vi "Update User Interface.vi"(8 "error in (no error)":errorcluster, 11 "Model in":refnum<class "Model.lvclass">) -> (0 "error out":errorcluster, 3 "Model out":refnum<class "Model.lvclass">)   [LabVIEW 2018, in "Model.lvlib" / "Model.lvclass"]
uses:
  Model.lvclass
  Model.lvclass/Model.ctl
  Interface Messages/Update VI List Msg/Update VI List Msg.lvclass/Update VI List Msg.ctl
  <vilib>/ActorFramework/Message Enqueuer/Message Enqueuer.lvclass/Message Enqueuer.ctl
  <vilib>/ActorFramework/Message Enqueuer/Enqueue.vi
  Interface Messages/Update VI List Msg/Update VI List Msg.lvclass
  C:/Program Files/National Instruments/LabVIEW 2018/vi.lib/ActorFramework/Message/Message.lvclass
  <vilib>/ActorFramework/Message Priority Queue/Priority Enqueue.vi
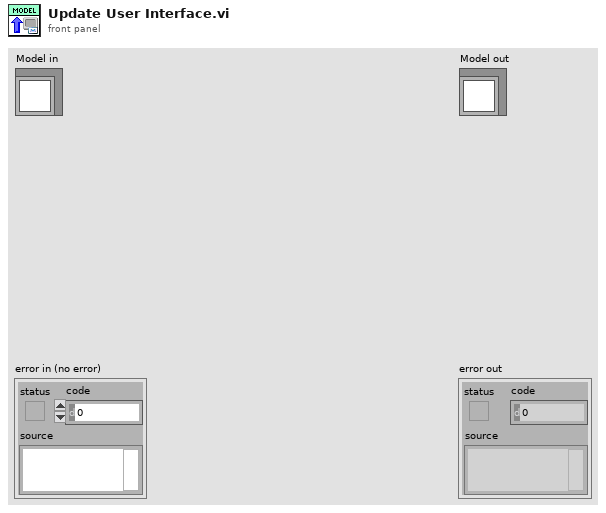
[diagram p1: front panel]
types:
  T1 = typedef "Model.lvlib/VI Infomation.ctl" = cluster{"Name":string, "Description":string, "Icon":picture}
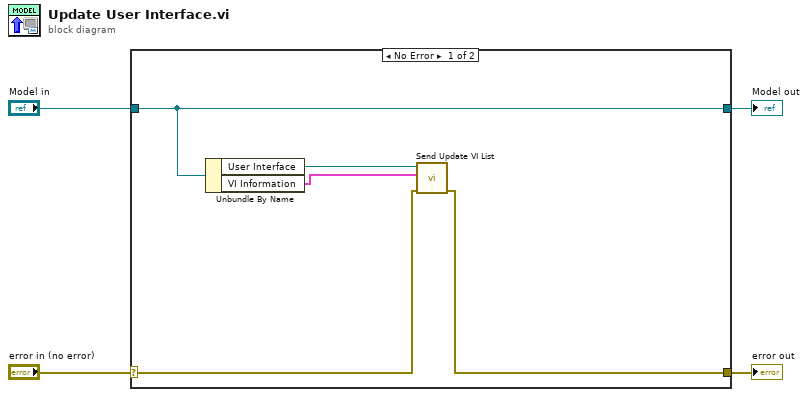
[diagram p0: block diagram]
diagram:
  n1 = case shown="No Error" "error in (no error)" {
    selector: "error in (no error)" -> [w6 w11]
    tunnel: [w5 w11] -> w3
    tunnel: [w9 w10] -> w1
    tunnel: "Model in" -> [w9 w10]
    frame No Error {
      n2 = Unbundle By Name(w9) -> ("User Interface"=w8:refnum<class "Message Enqueuer.lvclass">, "VI Information"=w7:T1[])
      n3 = call "Send Update VI List.vi"("error in (no error)"=w6, "VI Infomation"=w7, "Message Enqueuer"=w8) -> ("error out"=w5:errorcluster)  [unwired: 7 in, 1 out]
    }
    frame Error {
    }
  }
  "error out" <- w3
  "Model out" <- w1
